vi "Heartrate Monitor.vi"() -> ()   [LabVIEW 2017]
doc: "This VI acts as a heart rate monitor. It takes incoming voltage readings from a finger-clip heart-rate sensor and detects when there is a heart pulse (above 3 volts). It displays the voltage readings in real time on a waveform chart and keeps track of the number of pulses as well as the time elapsed. When stopped, the program outputs the average heart rate in beats/min."
panel:
  out "Heart Pulse Monitor":cluster{dbl, "Pulse":dbl}(graph)={4.84, "Pulse"=1.9316239316239316}
  in  "?":bool
  out "Heart Rate (beats/min)":dbl format="%#_2g"
  out "Elapsed Time (s)":dbl=4.84 format="%<%M:%S%2u>t"
  out "Pulse":bool=TRUE
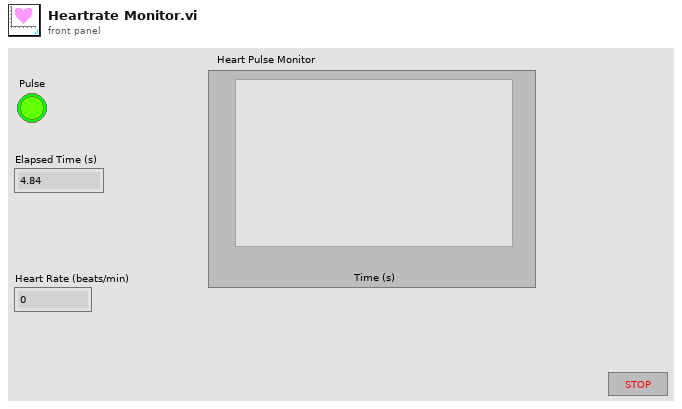
[diagram p1: front panel]
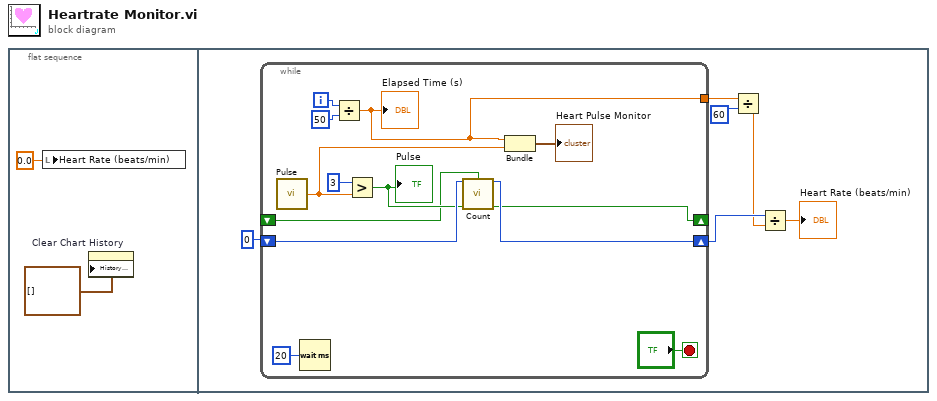
[diagram p0: block diagram]
diagram:
  n1 = flat-sequence {
    frame #0 {
      n2 = local write "Heart Rate (beats/min)"(0.0 ("Heart Rate (beats/min)")) -> ()
      n3 = property on="Clear Chart History" class="WFChart (strict)"("History Data"=cluster{dbl, "Pulse":dbl}[] []) -> ()  [unwired: 2 in, 2 out]
    }
    frame #1 {
      n4 = while {
        shift-right: [w15] -> w5
        shift-left: 0 -> [w16]
        tunnel: [w11] -> w7
        shift-right: [w13] -> _
        shift-left: _ -> [w12]
        i -> [w18]
        stop <- "?" stop-if-true
        n5 = call "Pulse.vi"() -> ("Pulse"=w10:dbl)  [unwired: 15 in]
        n6 = Wait (ms)(milliseconds to wait=u32 20) -> ()  [unwired: 1 out]
        n7 = Divide(x=w18, y=50) -> (x/y=w11:dbl)
        "Elapsed Time (s)" <- w11
        n8 = Greater?(x=3, y=w10) -> (0:w14:bool)
        "Pulse" <- w14
        n9 = call "Count.vi"("Start Count (SR)"=w16, "Switch"=w12, "Boolean In (SR)"=w14) -> ("Count (SR)"=w15:i32, "Boolean Out (SR)"=w13:bool)  [unwired: 11 in]
        n10 = Bundle(w11, "Pulse"=w10) -> (→"Heart Pulse Monitor":cluster{dbl, "Pulse":dbl})  [unwired: 1 in]
      }
      n11 = Divide(x=w7, y=60) -> (x/y=w4:dbl)
      n12 = Divide(x=w5, y=w4) -> (x/y=→"Heart Rate (beats/min)":dbl)
    }
  }
